vi "Parse CO2.vi"(6 "Processed Variables":T2 {"Chamber Temperature" format="%.2f"; "Ambient Temperature" format="%.2f"; "Bath Temperature" format="%.2f"; "Det. Temperature" format="%.2f"; "Detector Chl 4" format="%.2g"; "Detector Chl 3" format="%.2g"; "Ref CO2" format="%.2g"; "Detector Chl 2" format="%.2g"; "Film Temperature" format="%.2f"; "Humidity" format="%.2f"; "Detector Chl 1" format="%.2g"}, 10 "Daq Needed":T3 {"Current Settings"."Pump" items=["Pump 0", "Pump 1", "Pump 2", "Pump 3", "Pump 4", "Pump 5"]; "Current Settings"."Chart X axis Timescale" min=20 max=180 step=1; "Current Settings"."RunTime Mode Settings"."Exp. Gas Tank" items=["0.07", "0.031", "0.877", "1.863", "3.881", "5.790", "7.688", "6.000"]; "Current Settings"."RunTime Mode Settings"."Insp. Gas Tank" items=["0.07", "0.031", "0.877", "1.863", "3.881", "5.790", "7.688", "6.000"]; "Current Settings"."RunTime Mode Settings"."I:E Ratio" max=30 scale=0.0..7.0; "Current Settings"."RunTime Mode Settings"."Resp Rate Brpm" min=0 max=30 format="%.2f"; "Current Settings"."TE#2 Configuration"."Serial Port"."XOFF Char" format="%.0x"; "Current Settings"."TE#2 Configuration"."Serial Port"."XON Char" format="%.0x"; "Current Settings"."TE#2 Configuration"."Serial Port"."flow control" items=["None"=0, "XON/XOFF"=1, "RTS/CTS"=2, "DTR/DSR"=4]; "Current Settings"."TE#2 Configuration"."Serial Port"."stop bits" items=["1.0"=10, "1.5"=15, "2.0"=20]; "Current Settings"."TE#2 Configuration"."Serial Port"."data bits" min=5 max=8 step=1; "Current Settings"."TE#2 Configuration"."Serial Port"."baud rate" items=["75"=75, "110"=110, "134"=134, "150"=150, "300"=300, "600"=600, "1200"=1200, "1800"=1800, "2400"=2400, "4800"=4800, "7200"=7200, "9600"=9600, "14400"=14400, "19200"=19200, "28800"=28800, "38400"=38400, "56000"=56000, "57600"=57600, "115200"=115200, "128000"=128000, "230400"=230400]; "Current Settings"."TE#2 Configuration"."Serial Port"."termination char" format="%.0x"; "Current Settings"."TE#1 Configuration"."Serial Port"."XOFF Char" format="%.0x"; "Current Settings"."TE#1 Configuration"."Serial Port"."XON Char" format="%.0x"; "Current Settings"."TE#1 Configuration"."Serial Port"."flow control" items=["None"=0, "XON/XOFF"=1, "RTS/CTS"=2, "DTR/DSR"=4]; "Current Settings"."TE#1 Configuration"."Serial Port"."stop bits" items=["1.0"=10, "1.5"=15, "2.0"=20]; "Current Settings"."TE#1 Configuration"."Serial Port"."data bits" min=5 max=8 step=1; "Current Settings"."TE#1 Configuration"."Serial Port"."baud rate" items=["75"=75, "110"=110, "134"=134, "150"=150, "300"=300, "600"=600, "1200"=1200, "1800"=1800, "2400"=2400, "4800"=4800, "7200"=7200, "9600"=9600, "14400"=14400, "19200"=19200, "28800"=28800, "38400"=38400, "56000"=56000, "57600"=57600, "115200"=115200, "128000"=128000, "230400"=230400]; "Current Settings"."TE#1 Configuration"."Serial Port"."termination char" format="%.0x"; "Current Settings"."Capnometer Configuration"."Device" items=["None", "TidalWave", "LoFlow / Canary", "Capnogard"]; "Current Settings"."Capnometer Configuration"."Serial Port"."XOFF Char" format="%.0x"; "Current Settings"."Capnometer Configuration"."Serial Port"."XON Char" format="%.0x"; "Current Settings"."Capnometer Configuration"."Serial Port"."flow control" items=["None"=0, "XON/XOFF"=1, "RTS/CTS"=2, "DTR/DSR"=4]; "Current Settings"."Capnometer Configuration"."Serial Port"."stop bits" items=["1.0"=10, "1.5"=15, "2.0"=20]; "Current Settings"."Capnometer Configuration"."Serial Port"."data bits" min=5 max=8 step=1; "Current Settings"."Capnometer Configuration"."Serial Port"."baud rate" items=["75"=75, "110"=110, "134"=134, "150"=150, "300"=300, "600"=600, "1200"=1200, "1800"=1800, "2400"=2400, "4800"=4800, "7200"=7200, "9600"=9600, "14400"=14400, "19200"=19200, "28800"=28800, "38400"=38400, "56000"=56000, "57600"=57600, "115200"=115200, "128000"=128000, "230400"=230400]; "Current Settings"."Capnometer Configuration"."Serial Port"."termination char" format="%.0x"; "Current Settings"."DAQx Settings"."Analog Output Settings (Volts)" format="%#.3g"; "Current Settings"."DAQx Settings"."Duty Cycle" min=10.0 max=90.0 format="%.1g"; "Current Settings"."DAQx Settings"."Frequency" min=20.0 max=200.0; "Current Settings"."DataLogging Settings"."Data File Duration (Minutes)" min=2 max=200 format="%#.2g"; "Current Settings"."Calibration Settings"."Tolerance #2" min=2 max=4096; "Current Settings"."Calibration Settings"."Cal. Average" min=2 max=4096; "Current Settings"."Test Settings"."Test Sensor ID" items=["(select)", "RB", "YC", "", "Other"]}) -> (3 "Ticks Interval Time":dbl=200.0, 5 "output cluster":T1)   [LabVIEW 2016]
uses:
  Controls/DAQ Needed.ctl
  Controls/Processed Variables.ctl
  Controls/AirPump Controls.ctl
  Controls/IE Ratio knob.ctl
  Controls/UI Settings.ctl
  Controls/Aux CO2 Control.ctl
  Controls/Serial Visa Control.ctl
  Controls/Aux CO2 Selector.ctl
  Controls/Aux TE Control.ctl
  Controls/Queues And Others.ctl
panel:
  out "x > 0?":bool
  # "Note: Setting Brpm to zero will\ndisable Insp / Exp digital output."
  # "mmHg"
  # "pts"
  # "tolerance"
  # "AN5 (Temp 1)"
  # "AN6 (Temp 2)"
  # "AN7 (Temp 3)"
  # "AN8 (T FET)"
  # "AN0 (T POT)"
  # "Tref (Set Pt))"
  # "(Spare)"
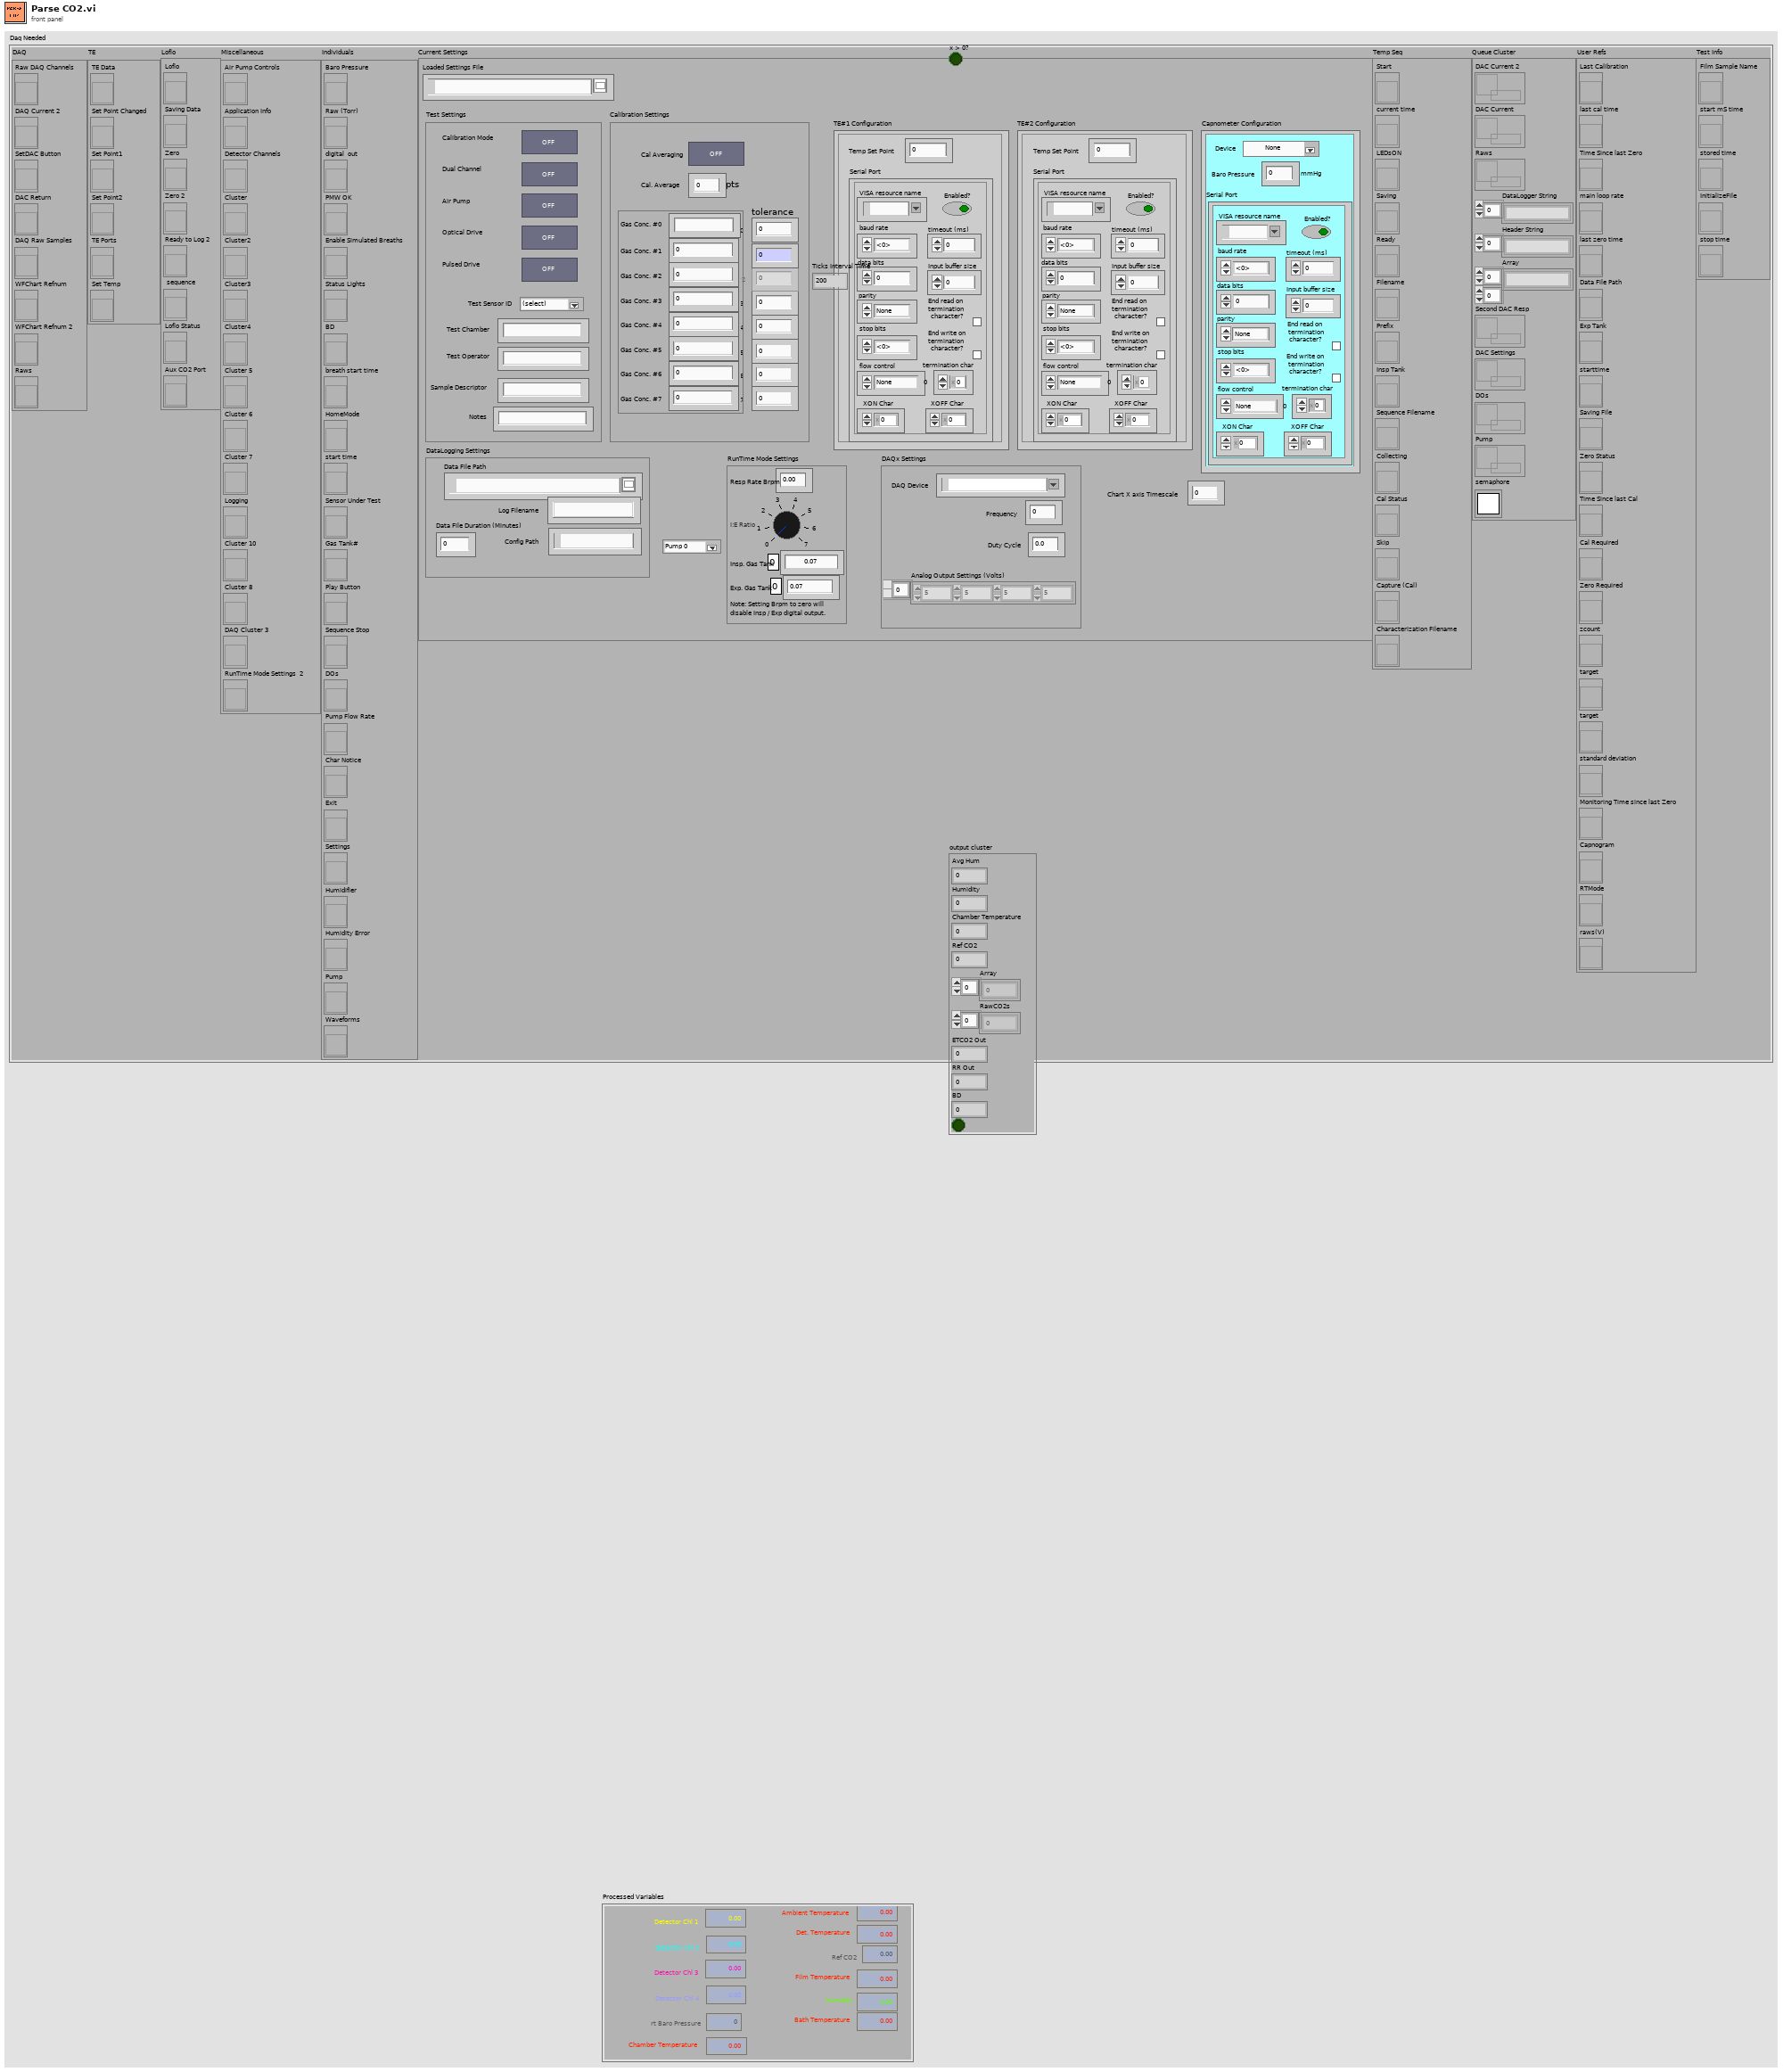
[diagram p1: front panel]
types:
  T1 = cluster{"Avg Hum":dbl, "Humidity":dbl, "Chamber Temperature":dbl, "Ref CO2":sgl, "Array":sgl[], "RawCO2s":dbl[], "ETCO2 Out":dbl, "RR Out":dbl, "BD":i32, bool}
  T2 = typedef "Processed Variables.ctl" = cluster{"Detector Chl 1":sgl, "Humidity":dbl, "Film Temperature":dbl, "Detector Chl 2":sgl, "Ref CO2":sgl, "Detector Chl 3":sgl, "Detector Chl 4":sgl, "Det. Temperature":dbl, "Bath Temperature":dbl, "Ambient Temperature":dbl, "rt Baro Pressure":u16, "Chamber Temperature":dbl}
  T3 = typedef "DAQ Needed.ctl" = cluster{"DAQ":cluster{"Raw DAQ Channels":refnum<vi>, "DAQ Current 2":refnum<vi>, "SetDAC Button":refnum<vi>, "DAC Return":refnum<vi>, "DAQ Raw Samples":refnum<vi>, "WFChart Refnum":refnum<vi>, "WFChart Refnum 2":refnum<vi>, "Raws":refnum<vi>}, "TE":cluster{"TE Data":refnum<vi>, "Set Point Changed":refnum<vi>, "Set Point1":refnum<vi>, "Set Point2":refnum<vi>, "TE Ports":refnum<vi>, "Set Temp":refnum<vi>}, "Loflo":cluster{"Loflo":refnum<vi>, "Saving Data":refnum<vi>, "Zero":refnum<vi>, "Zero 2":refnum<vi>, "Ready to Log 2":refnum<vi>, " sequence":refnum<vi>, "Loflo Status ":refnum<vi>, "Aux CO2 Port":refnum<vi>}, "Miscellaneous":cluster{"Air Pump Controls":refnum<vi>, "Application Info":refnum<vi>, "Detector Channels ":refnum<vi>, "Cluster":refnum<vi>, "Cluster2":refnum<vi>, "Cluster3":refnum<vi>, "Cluster4":refnum<vi>, "Cluster 5":refnum<vi>, "Cluster 6":refnum<vi>, "Cluster 7":refnum<vi>, "Logging":refnum<vi>, "Cluster 10":refnum<vi>, "Cluster 8":refnum<vi>, "DAQ Cluster 3":refnum<vi>, "RunTime Mode Settings  2":refnum<vi>}, "Individuals":cluster{"Baro Pressure":refnum<vi>, "Raw (Torr)":refnum<vi>, "digital  out":refnum<vi>, "PMW OK":refnum<vi>, "Enable Simulated Breaths":refnum<vi>, "Status Lights":refnum<vi>, "BD":refnum<vi>, "breath start time":refnum<vi>, "HomeMode":refnum<vi>, "start time":refnum<vi>, "Sensor Under Test":refnum<vi>, "Gas Tank#":refnum<vi>, "Play Button":refnum<vi>, "Sequence Stop":refnum<vi>, "DOs":refnum<vi>, "Pump Flow Rate":refnum<vi>, "Char Notice":refnum<vi>, "Exit":refnum<vi>, "Settings":refnum<vi>, "Humidifier":refnum<vi>, "Humidity Error":refnum<vi>, "Pump":refnum<vi>, "Waveforms":refnum<vi>}, "Current Settings":T4, "Temp Seq":cluster{"Start":refnum<vi>, "current time":refnum<vi>, "LEDsON":refnum<vi>, "Saving":refnum<vi>, "Ready":refnum<vi>, "Filename":refnum<vi>, "Prefix":refnum<vi>, "Insp Tank":refnum<vi>, "Sequence Filename":refnum<vi>, "Collecting":refnum<vi>, "Cal Status":refnum<vi>, "Skip":refnum<vi>, "Capture (Cal)":refnum<vi>, "Characterization Filename":refnum<vi>}, "Queue Cluster":T9, "User Refs":cluster{"Last Calibration":refnum<vi>, "last cal time":refnum<vi>, "Time Since last Zero":refnum<vi>, "main loop rate":refnum<vi>, "last zero time":refnum<vi>, "Data File Path":refnum<vi>, "Exp Tank":refnum<vi>, "starttime":refnum<vi>, "Saving File":refnum<vi>, "Zero Status":refnum<vi>, "Time Since last Cal":refnum<vi>, "Cal Required":refnum<vi>, "Zero Required":refnum<vi>, "zcount":refnum<vi>, "target":refnum<vi>, "target":refnum<vi>, "standard deviation":refnum<vi>, "Monitoring Time since last Zero":refnum<vi>, "Capnogram":refnum<vi>, "RTMode":refnum<vi>, "raws(V)":refnum<vi>}, "Test Info":cluster{"Film Sample Name":refnum<vi>, "start mS time":refnum<vi>, "stored time":refnum<vi>, "InitializeFile":refnum<vi>, "stop time":refnum<vi>}}
  T4 = typedef "UI Settings.ctl" = cluster{"Loaded Settings File":path, "Test Settings":cluster{"Dual Channel":bool, "Air Pump":bool, "Optical Drive":bool, "Pulsed Drive":bool, "Calibration Mode":bool, "Test Sensor ID":u16, "Test Chamber":string, "Test Operator":string, "Sample Descriptor":string, "Notes":string}, "Calibration Settings":cluster{"Cal. Average":u16, "Cal Averaging":bool, "Tolerance #0":sgl, "Tolerance #7":sgl, "Tolerance #6":sgl, "Tolerance #5":sgl, "Tolerance #4":sgl, "Tolerance #3":sgl, "Tolerance #2":sgl, "Tolerance #1":sgl, "Gas Tank Settings":cluster{"Gas Conc. #0":string, "Gas Conc. #1":sgl, "Gas Conc. #2":sgl, "Gas Conc. #3":sgl, "Gas Conc. #4":sgl, "Gas Conc. #5":sgl, "Gas Conc. #6":sgl, "Gas Conc. #7":sgl}}, "DataLogging Settings":cluster{"Data File Path":path, "Data File Duration (Minutes)":sgl, "Log Filename":string, "Config Path":path}, "DAQx Settings":cluster{"DAQ Device":tag, "Frequency":dbl, "Duty Cycle":dbl, "Analog Output Settings (Volts)":sgl[]}, "Capnometer Configuration":T5, "TE#1 Configuration":T8, "TE#2 Configuration":T8, "RunTime Mode Settings ":cluster{"Resp Rate Brpm ":sgl, "I:E Ratio":u8, "Insp. Gas Tank":u16, "Exp. Gas Tank":u16}, "Chart X axis Timescale":u16, "Pump":u16}
  T5 = typedef "Aux CO2 Control.ctl" = cluster{"Serial Port":T6, "Baro Pressure":u32, "Device":T7}
  T6 = typedef "Serial Visa Control.ctl" = cluster{"termination char":u8, "End read on termination character?":bool, "Enabled?":bool, "VISA resource name":refnum<visa-resource-name>, "baud rate":u32, "data bits":u16, "parity":enum16{"None", "Odd", "Even", "Mark", "Space"}, "stop bits":u16, "flow control":u16, "timeout (ms)":u32, "Input buffer size":u32, "End write on termination character?":bool, "XON Char":u8, "XOFF Char":u8}
  T7 = typedef "Aux CO2 Selector.ctl" = u16
  T8 = typedef "Aux TE Control.ctl" = cluster{"Temp Set Point":sgl, "Serial Port":T6}
  T9 = typedef "Queues And Others.ctl" = cluster{"DAC Current 2":refnum<queue>, "DAC Current":refnum<queue>, "Raws":refnum<queue>, "DataLogger String":string[], "Header String":string[], "Array":string[][], "Second DAC Resp":refnum<queue>, "DAC Settings":refnum<queue>, "DOs":refnum<queue>, "Pump":refnum<queue>, "semaphore":T10}
  T10 = typedef "Semaphore RefNum" = refnum<k1>
  T11 = cluster{"Avg_Hum":sgl, "Humidity":dbl, "Chamber Temperature":dbl, "Ref CO2":sgl, "Array":sgl[], "RawCO2s":dbl[], "ETCO2 Out":dbl, "RR Out":dbl, "BD":i32, "x>0":bool}
  T12 = cluster{"ETCO2 %":sgl, "RR (brpm)":sgl, "Inhale Time":sgl, "Exhale Time":sgl, "Enable Simulated Breaths":bool, "Use Channel":u8}
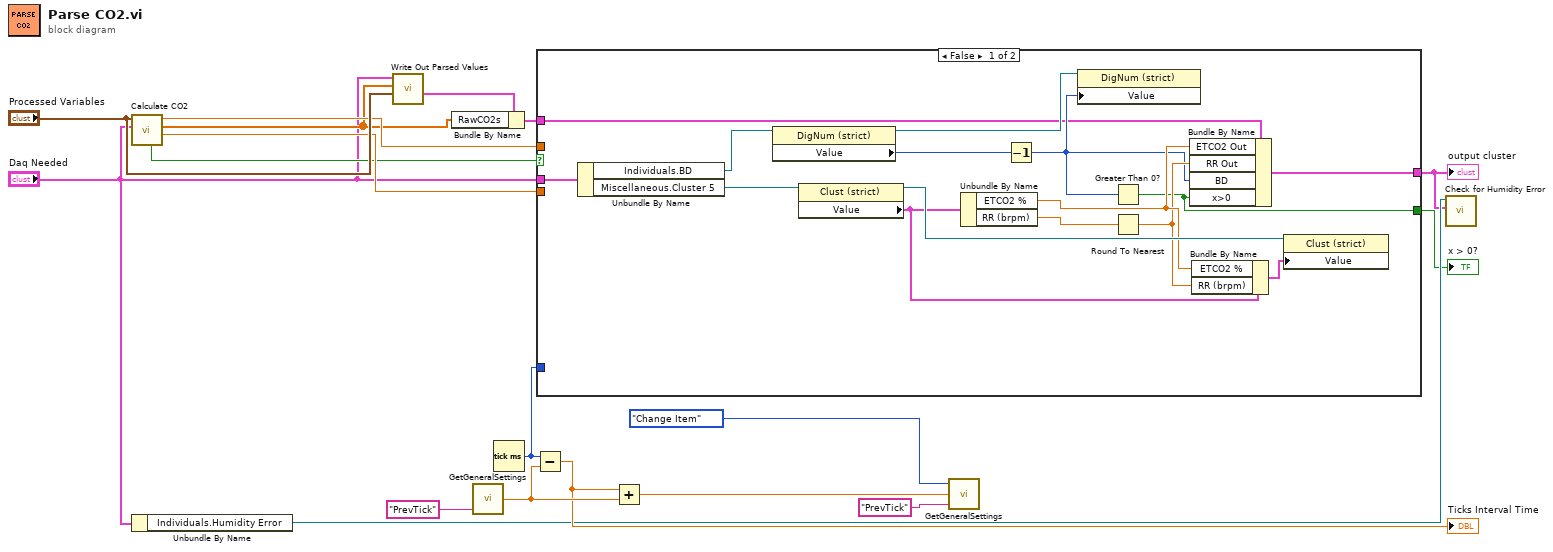
[diagram p0: block diagram]
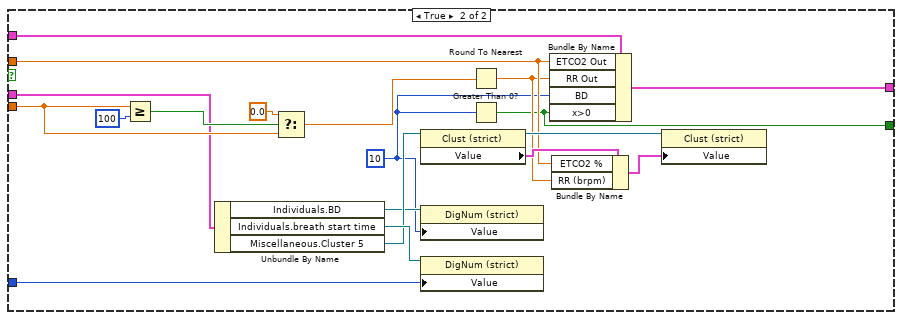
[diagram p2: hidden frame]
diagram:
  n1 = call "Calculate CO2.vi"("Daq Needed"="Daq Needed", "Processed Variables"="Processed Variables") -> ("RR Out"=w17:dbl, "Raws"=w8:sgl[], "ETCO2 Out"=w16:dbl, "New Breath Found"=w15:bool)  [unwired: 6 in]
  n2 = Unbundle By Name("Daq Needed") -> ("Individuals.Humidity Error"=w6:refnum<vi>)
  n3 = call "Write Out Parsed Values.vi"("Processed Variables"="Processed Variables", "RawCO2s"=w8, "Daq Needed"="Daq Needed") -> ("output cluster"=w4:T11)  [unwired: 4 in, 4 out]
  n4 = Bundle By Name(cluster=w4, "RawCO2s"=w8) -> (w2:T11)
  n5 = call "GetGeneralSettings.vi"("Variable Name"="PrevTick") -> ("Set Value"=w10:dbl)  [unwired: 2 in]
  n6 = Tick Count (ms)() -> (millisecond timer value=w7:u32)
  n7 = Subtract(x=w7, y=w10) -> (x-y=w9:dbl)
  "Ticks Interval Time" <- w9
  n8 = case shown="False" w15 {
    tunnel: w16 -> [_ w39]
    tunnel: w17 -> [_ w51]
    tunnel: w7 -> [_ w48]
    tunnel: "Daq Needed" -> [w28 w43]
    tunnel: [w21 w36] -> w3
    tunnel: w2 -> [w20 w35]
    tunnel: [w19 w34] -> w1
    frame False {
      n9 = Unbundle By Name(w28) -> ("Individuals.BD"=w27:refnum<vi>, "Miscellaneous.Cluster 5"=w26:refnum<vi>)
      n10 = property class="DigNum (strict)"(reference=w27) -> (reference out=w25:refnum<vi>, "Value"=w33:i32)  [unwired: 1 in, 1 out]
      n11 = property class="Clust (strict)"(reference=w26) -> (reference out=w32:refnum<vi>, "Value"=w31:T12)  [unwired: 1 in, 1 out]
      n12 = Unbundle By Name(w31) -> ("ETCO2 %"=w24:sgl, "RR (brpm)"=w29:sgl)
      n13 = Decrement(x=w33) -> (x-1=w22:i32)
      n14 = property class="DigNum (strict)"(reference=w25, "Value"=w22) -> ()  [unwired: 1 in, 2 out]
      n15 = Greater Than 0?(x=w22) -> (x > 0?=w21:bool)
      n16 = Round To Nearest(number=w29) -> (nearest integer value=w23:sgl)
      n17 = Bundle By Name(cluster=w20, "ETCO2 Out"=w24, "RR Out"=w23, "BD"=w22, "x>0"=w21) -> (w19:T11)
      n18 = Bundle By Name(cluster=w31, "ETCO2 %"=w24, "RR (brpm)"=w23) -> (w30:T12)
      n19 = property class="Clust (strict)"(reference=w32, "Value"=w30) -> ()  [unwired: 1 in, 2 out]
    }
    frame True {
      w37 = u8 10 ("BD")
      n20 = Greater Or Equal?(x=w51, y=100) -> (x >= y?=w50:bool)
      n21 = Unbundle By Name(w43) -> ("Individuals.BD"=w40:refnum<vi>, "Individuals.breath start time"=w42:refnum<vi>, "Miscellaneous.Cluster 5"=w41:refnum<vi>)
      n22 = Select(t=0.0, s=w50, f=w51) -> (s? t:f=w44:dbl)
      n23 = property class="Clust (strict)"(reference=w41) -> (reference out=w46:refnum<vi>, "Value"=w47:T12)  [unwired: 1 in, 1 out]
      n24 = property class="DigNum (strict)"(reference=w40, "Value"=w37) -> ()  [unwired: 1 in, 2 out]
      n25 = property class="DigNum (strict)"(reference=w42, "Value"=w48) -> ()  [unwired: 1 in, 2 out]
      n26 = Round To Nearest(number=w44) -> (nearest integer value=w38:dbl)
      n27 = Greater Than 0?(x=w37) -> (x > 0?=w36:bool)
      n28 = Bundle By Name(cluster=w35, "ETCO2 Out"=w39, "RR Out"=w38, "BD"=w37, "x>0"=w36) -> (w34:T11)
      n29 = Bundle By Name(cluster=w47, "ETCO2 %"=w39, "RR (brpm)"=w38) -> (w45:T12)
      n30 = property class="Clust (strict)"(reference=w46, "Value"=w45) -> ()  [unwired: 1 in, 2 out]
    }
  }
  "x > 0?" <- w3
  "output cluster" <- w1
  n31 = Add(x=w9, y=w10) -> (x+y=w12:dbl)
  n32 = call "GetGeneralSettings.vi"("Variable Name"="PrevTick", "Change Value"=w12, "Mode"=enum16{"Change Item", "Get Value"}."Change Item") -> ()  [unwired: 1 out]
  n33 = call "Check for Humidity Error.vi"("output cluster"=w1, "Boolean in"=w6) -> ()  [unwired: 9 in, 1 out]
